vi "Tree Column Header.vi"(0 "[V]System Tree View in":refnum<class "[V]System Tree View.lvclass">, 1 "Style":T1={"Bold"=TRUE, "Justification"=enum."Left", "Font:Size"=18, "Font:Color"=15856113, "BG Color"=1752220}, 5 "Header Width Ratio":dbl[](array[numeric])=[0.5, 0.1], 7 "Header Names":string[](array[string])=["File", " "], 11 "error in (no error)":errorcluster) -> (4 "[V]System Tree View out":refnum<class "[V]System Tree View.lvclass">, 15 "error out":errorcluster)   [LabVIEW 2020, in "[V]System Tree View.lvlib" / "[V]System Tree View.lvclass"]
uses:
  [V]System Tree View.lvclass
  [V]System Tree View.lvclass/[V]System Tree View.ctl
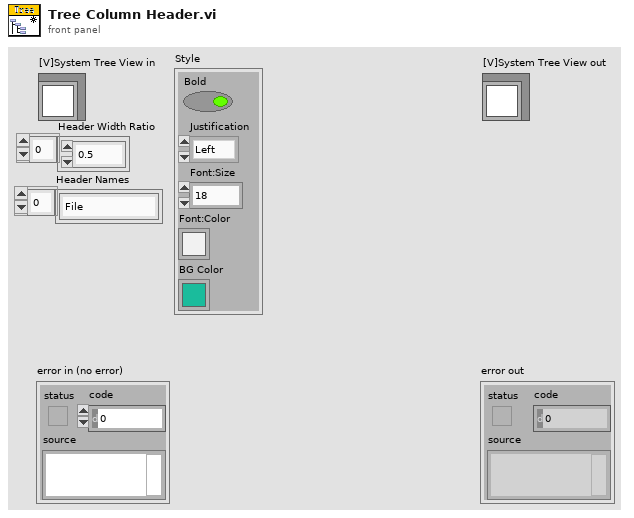
[diagram p1: front panel]
types:
  T1 = cluster{"Bold":bool, "Justification":enum16{"Left", "Center", "Right"}, "Font:Size":u32, "Font:Color":u32, "BG Color":u32}
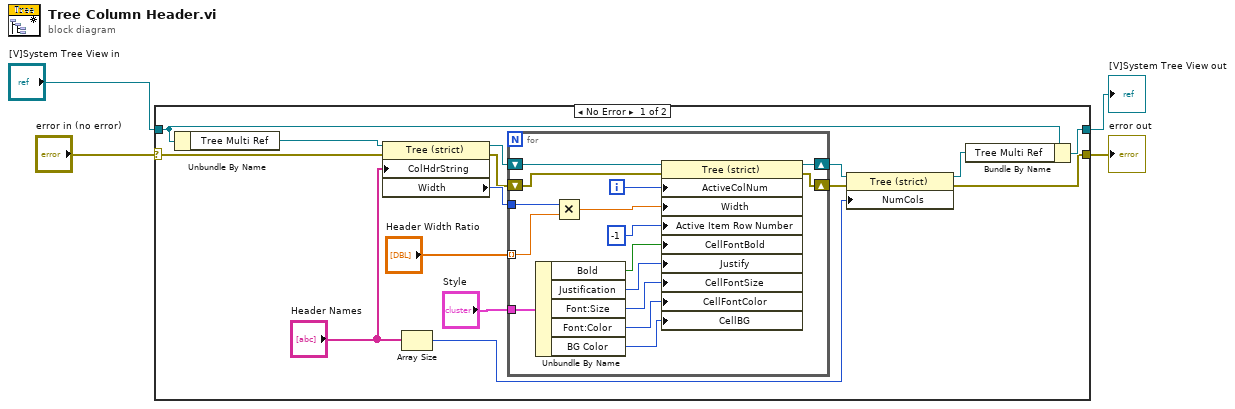
[diagram p0: block diagram]
diagram:
  n1 = case shown="No Error" "error in (no error)" {
    selector: "error in (no error)" -> [w6 w36]
    tunnel: [w5 w36] -> w3
    tunnel: [w18 w35] -> w1
    tunnel: "[V]System Tree View in" -> [w19 w35]
    frame No Error {
      n2 = Unbundle By Name(w19) -> ("Tree Multi Ref"=w17:refnum<vi>)
      n3 = property class="Tree (strict)"(reference=w17, error in=w6, "ColHdrString"="Header Names") -> (reference out=w14:refnum<vi>, error out=w10:errorcluster, "Width"=w15:u32)
      n4 = Array Size(array="Header Names") -> (size(s)=w8:i32)
      n5 = for {
        tunnel: "Header Width Ratio" -> [w30] mode=indexing
        tunnel: w15 -> [w31]
        shift-right: [w33] -> w11
        shift-left: w14 -> [w34]
        tunnel: "Style" -> [w27]
        shift-right: [w21] -> w9
        shift-left: w10 -> [w20]
        i -> [w32]
        n6 = Unbundle By Name(w27) -> ("Bold"=w26:bool, "Justification"=w25:enum16{"Left", "Center", "Right"}, "Font:Size"=w24:u32, "Font:Color"=w23:u32, "BG Color"=w22:u32)
        n7 = Multiply(x=w31, y=w30) -> (x*y=w29:dbl)
        n8 = property class="Tree (strict)"(reference=w34, error in=w20, "ActiveColNum"=w32, "Width"=w29, "Active Item Row Number"=-1 ("Active Item:Row Number"), "CellFontBold"=w26, "Justify"=w25, "CellFontSize"=w24, "CellFontColor"=w23, "CellBG"=w22) -> (reference out=w33:refnum<vi>, error out=w21:errorcluster)
      }
      n9 = property class="Tree (strict)"(reference=w11, error in=w9, "NumCols"=w8) -> (reference out=w7:refnum<vi>, error out=w5:errorcluster)
      n10 = Bundle By Name(cluster=w19, "Tree Multi Ref"=w7) -> (w18:refnum<class "[V]System Tree View.lvclass">)
    }
    frame Error {
    }
  }
  "error out" <- w3
  "[V]System Tree View out" <- w1
